vi "Base64url_CharSet.vi"() -> (3 "base64 URL charset":u8[](array[numeric]))   [LabVIEW 2017, in "Serializer.Base64.lvclass"]
uses:
  Serializer.Base64.lvclass
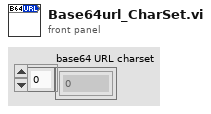
[diagram p1: front panel]
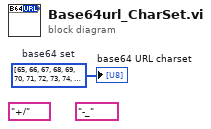
[diagram p0: block diagram]
diagram:
  (unwired) "-_"
  (unwired) "+/"
  w1 = u8[] [65, 66, 67, 68, 69, 70, 71, 72, 73, 74, 75, 76, 77, 78, 79, 80, 81, 82, 83, 84, 85, 86, 87, 88, 89, 90, 97, 98, 99, 100, 101, 102, 103, 104, 105, 106, 107, 108, 109, 110, 111, 112, 113, 114, 115, 116, 117, 118, 119, 120, 121, 122, 48, 49, 50, 51, 52, 53, 54, 55, 56, 57, 45, 95]  # base64 set
  "base64 URL charset" <- w1
